vi "Receive Starter Kit Message.vi"(8 "error in (no error)":errorcluster, 9 "timeout ms (25000)":i32, 11 "connection ID in":refnum<k5>) -> (0 "error out":errorcluster, 2 "message":T1={"message type"=enum."Motor Vel SP", "message data"=variant}, 3 "connection ID out":refnum<k5>)   [LabVIEW 2010]
uses:
  Starter Kit Message.ctl
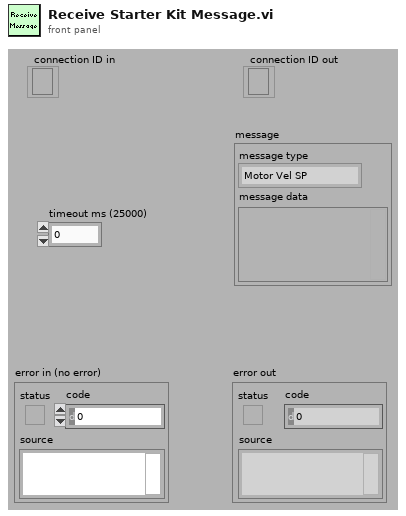
[diagram p1: front panel]
types:
  T1 = typedef "Starter Kit Message.ctl" = cluster{"message type":enum16{"Heartbeat", "Motor Vel SP", "Servo Angle", "Stop"}, "message data":variant}
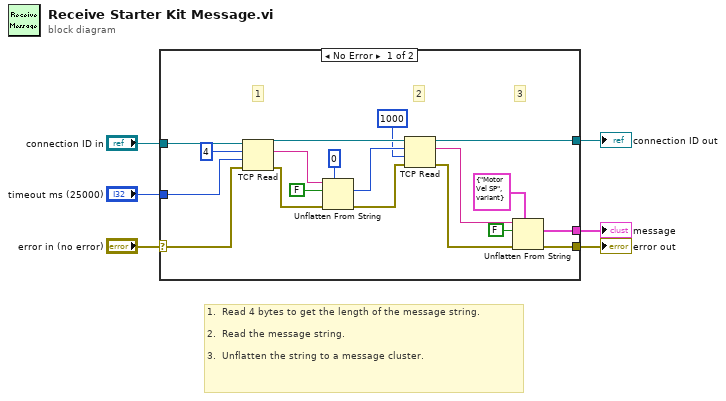
[diagram p0: block diagram]
diagram:
  # "1.  Read 4 bytes to get the length of the message string.\n\n2.  Read the message string.\n\n3.  Unflatten the string to a message cluster."
  n1 = case shown="No Error" "error in (no error)" {
    selector: "error in (no error)" -> [w7 w27]
    tunnel: "connection ID in" -> [w17 w26]
    tunnel: [w14 w26] -> w5
    tunnel: [w11 _] -> w4
    tunnel: "timeout ms (25000)" -> [w10 _]
    tunnel: [w8 w27] -> w1
    frame No Error {
      # "3"
      # "2"
      # "1"
      n2 = TCP Read(connection ID=w17, bytes to read=4, error in (no error)=w7, 9:w10) -> (connection ID out=w19:refnum<k5>, data out=w21:string, error out=w24:errorcluster)  [unwired: 1 out]
      n3 = Unflatten From String(type=0, binary string=w21, data includes array or string size? (T)=FALSE, error in (no error)=w24) -> (value=w22:i32, error out=w25:errorcluster)  [unwired: 2 out]
      n4 = TCP Read(connection ID=w19, bytes to read=w22, error in (no error)=w25, 9:1000 ("timeout ms (25000)")) -> (connection ID out=w14:refnum<k5>, data out=w13:string, error out=w12:errorcluster)  [unwired: 1 out]
      n5 = Unflatten From String(type=T1 {"message type"=enum."Motor Vel SP", "message data"=variant} ("message"), binary string=w13, data includes array or string size? (T)=FALSE, error in (no error)=w12) -> (value=w11:T1, error out=w8:errorcluster)  [unwired: 2 out]
    }
    frame Error {
    }
  }
  "connection ID out" <- w5
  "message" <- w4
  "error out" <- w1
